vi "LocalTimeString.vi"(4 "Time Stamp":timestamp) -> (1 "Local Time String":string)   [LabVIEW 2015, in "DBToolkit.lvlib"]
uses:
  DBToolkit.lvlib
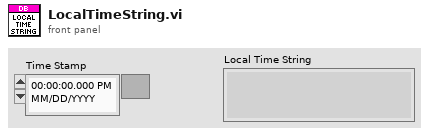
[diagram p1: front panel]
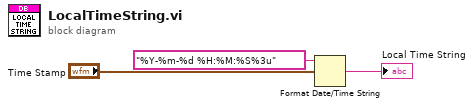
[diagram p0: block diagram]
diagram:
  n1 = Format Date/Time String(time format string (%c)="%Y-%m-%d %H:%M:%S%3u", seconds (now)="Time Stamp") -> (date/time string=→"Local Time String":string)  [unwired: 1 in]
